vi "Layer_Poly.vi"   [LabVIEW 2018]
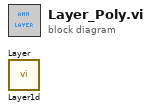
[diagram p0: block diagram]
diagram:
  n1 = call "Layer1d.vi"() -> ()  [unwired: 9 in, 3 out]
  n2 = call "Layer.vi"() -> ()  [unwired: 9 in, 3 out]
